vi "fgv_AOL Properties.vi"(8 "error in (no error)":errorcluster, 10 "Function":T2, 11 "AOL Properties in":T1={"AOD 1 thickness (mm)"=118.0, "AOD 2 thickness (mm)"=115.0, "AOD 3 thickness (mm)"=110.0, "AOD 4 thickness (mm)"=135.0, "AOD 5 thickness (mm)"=135.0, "AOD 6 thickness (mm)"=135.0, "AOD 1-2 separation (mm)"=15.0, "AOD 2-3 separation (mm)"=15.0, "AOD 3-4 separation (mm)"=15.0, "AOD 4-5 separation (mm)"=15.0, "AOD 5-6 separation (mm)"=15.0, "AOD 1 X Offset"=15.0, "AOD 2 X Offset"=1.0, "AOD 3 X Offset"=1.0, "AOD 4 X Offset"=1.0, "AOD 1 Y Offset"=1.0, "AOD 2 Y Offset"=1.0, "AOD 3 Y Offset"=1.0, "AOD 4 Y Offset"=1.0, "AOD 1 X Direction"=0.0, "AOD 2 X Direction"=0.0, "AOD 3 X Direction"=0.0, "AOD 4 X Direction"=0.0, "AOD 1 Y Direction"=1.0, "AOD 2 Y Direction"=0.0, "AOD 3 Y Direction"=0.0023, "AOD 4 Y Direction"=0.0046, "AOD 1 Centre (mm)"=15.0, "AOD 2 Centre (mm)"=50.0, "AOD 3 Centre (mm)"=50.0, "AOD 4 Centre (mm)"=50.0, "Timing Offset AOD 1"=0.0, "Timing Offset AOD 2"=0.0, "Timing Offset AOD 3"=0.0, "Timing Offset AOD 4"=0.0, "AOD Optical offset 1"=20000.0, "AOD Optical offset 2"=20000.0, "AOL aperture (mm)"=15.0, "AOL centre wavelength (nm)"=1.0, "AOL centre frequency (MHz)"=1.0, "Diffraction mode"=1.0, "Crystal length (mm)"=0.0, "Acoustic velocity (m/s)"=1.0, "Pair deflection ratio"=1.0, "AOD fill time (us)"=1.0, "AOD Ord. Refractive index"=2.22, "AOD ExtraOrd. Refractive index"=2.22}) -> (0 "error out":errorcluster, 3 "AOL Properties out":T1={"AOD 1 thickness (mm)"=118.0, "AOD 2 thickness (mm)"=115.0, "AOD 3 thickness (mm)"=110.0, "AOD 4 thickness (mm)"=135.0, "AOD 5 thickness (mm)"=135.0, "AOD 6 thickness (mm)"=135.0, "AOD 1-2 separation (mm)"=15.0, "AOD 2-3 separation (mm)"=15.0, "AOD 3-4 separation (mm)"=15.0, "AOD 4-5 separation (mm)"=15.0, "AOD 5-6 separation (mm)"=15.0, "AOD 1 X Offset"=15.0, "AOD 2 X Offset"=1.0, "AOD 3 X Offset"=1.0, "AOD 4 X Offset"=1.0, "AOD 1 Y Offset"=1.0, "AOD 2 Y Offset"=1.0, "AOD 3 Y Offset"=1.0, "AOD 4 Y Offset"=1.0, "AOD 1 X Direction"=0.0, "AOD 2 X Direction"=0.0, "AOD 3 X Direction"=0.0, "AOD 4 X Direction"=0.0, "AOD 1 Y Direction"=1.0, "AOD 2 Y Direction"=0.0, "AOD 3 Y Direction"=0.0023, "AOD 4 Y Direction"=0.0046, "AOD 1 Centre (mm)"=15.0, "AOD 2 Centre (mm)"=50.0, "AOD 3 Centre (mm)"=50.0, "AOD 4 Centre (mm)"=50.0, "Timing Offset AOD 1"=0.0, "Timing Offset AOD 2"=0.0, "Timing Offset AOD 3"=0.0, "Timing Offset AOD 4"=0.0, "AOD Optical offset 1"=20000.0, "AOD Optical offset 2"=20000.0, "AOL aperture (mm)"=15.0, "AOL centre wavelength (nm)"=1.0, "AOL centre frequency (MHz)"=1.0, "Diffraction mode"=1.0, "Crystal length (mm)"=0.0, "Acoustic velocity (m/s)"=1.0, "Pair deflection ratio"=1.0, "AOD fill time (us)"=1.0, "AOD Ord. Refractive index"=2.22, "AOD ExtraOrd. Refractive index"=2.22})   [LabVIEW 2017]
uses:
  Typedefs/AOL Properties Cluster.ctl
  Typedefs/HW config states enum.ctl
  Typedefs/Save-Load enum.ctl
  General Globals.vi
panel:
  # "FUNCTIONAL GLOBAL"
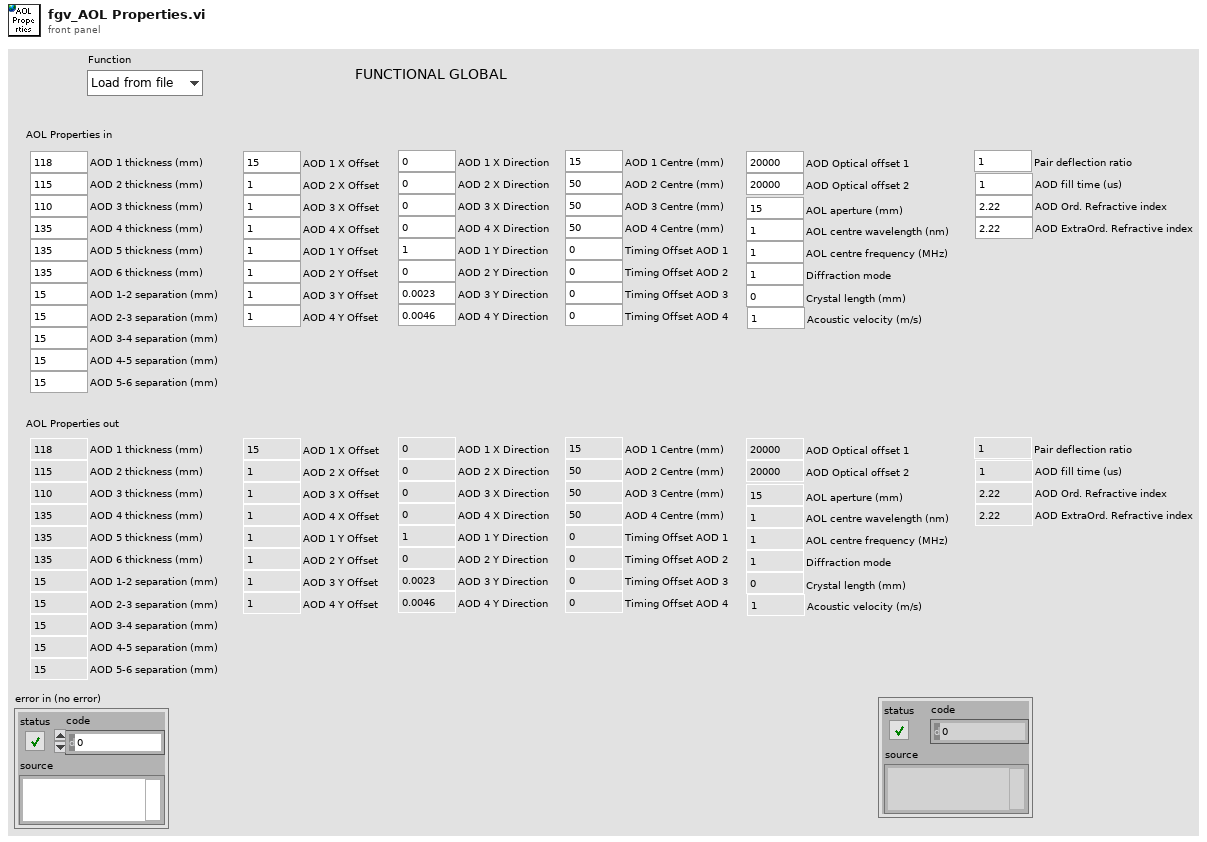
[diagram p1: front panel]
types:
  T1 = typedef "AOL Properties Cluster.ctl" = cluster{"AOD 1 thickness (mm)":dbl, "AOD 2 thickness (mm)":dbl, "AOD 3 thickness (mm)":dbl, "AOD 4 thickness (mm)":dbl, "AOD 5 thickness (mm)":dbl, "AOD 6 thickness (mm)":dbl, "AOD 1-2 separation (mm)":dbl, "AOD 2-3 separation (mm)":dbl, "AOD 3-4 separation (mm)":dbl, "AOD 4-5 separation (mm)":dbl, "AOD 5-6 separation (mm)":dbl, "AOD 1 X Offset":dbl, "AOD 2 X Offset":dbl, "AOD 3 X Offset":dbl, "AOD 4 X Offset":dbl, "AOD 1 Y Offset":dbl, "AOD 2 Y Offset":dbl, "AOD 3 Y Offset":dbl, "AOD 4 Y Offset":dbl, "AOD 1 X Direction":dbl, "AOD 2 X Direction":dbl, "AOD 3 X Direction":dbl, "AOD 4 X Direction":dbl, "AOD 1 Y Direction":dbl, "AOD 2 Y Direction":dbl, "AOD 3 Y Direction":dbl, "AOD 4 Y Direction":dbl, "AOD 1 Centre (mm)":dbl, "AOD 2 Centre (mm)":dbl, "AOD 3 Centre (mm)":dbl, "AOD 4 Centre (mm)":dbl, "Timing Offset AOD 1":dbl, "Timing Offset AOD 2":dbl, "Timing Offset AOD 3":dbl, "Timing Offset AOD 4":dbl, "AOD Optical offset 1":dbl, "AOD Optical offset 2":dbl, "AOL aperture (mm)":dbl, "AOL centre wavelength (nm)":dbl, "AOL centre frequency (MHz)":dbl, "Diffraction mode":dbl, "Crystal length (mm)":dbl, "Acoustic velocity (m/s)":dbl, "Pair deflection ratio":dbl, "AOD fill time (us)":dbl, "AOD Ord. Refractive index":dbl, "AOD ExtraOrd. Refractive index":dbl}
  T2 = typedef "HW config states enum.ctl" = enum16{"Load from file", "Save to file", "Write all", "Read all", "Write XY stage settings", "Write DAQ FPGA settings", "Write Control FPGA settings", "Write Phys Channels", "Clear", "Compare from file"}
  T3 = typedef "Save-Load enum.ctl" = enum16{"Save to file", "Load from file", "Compare from file"}
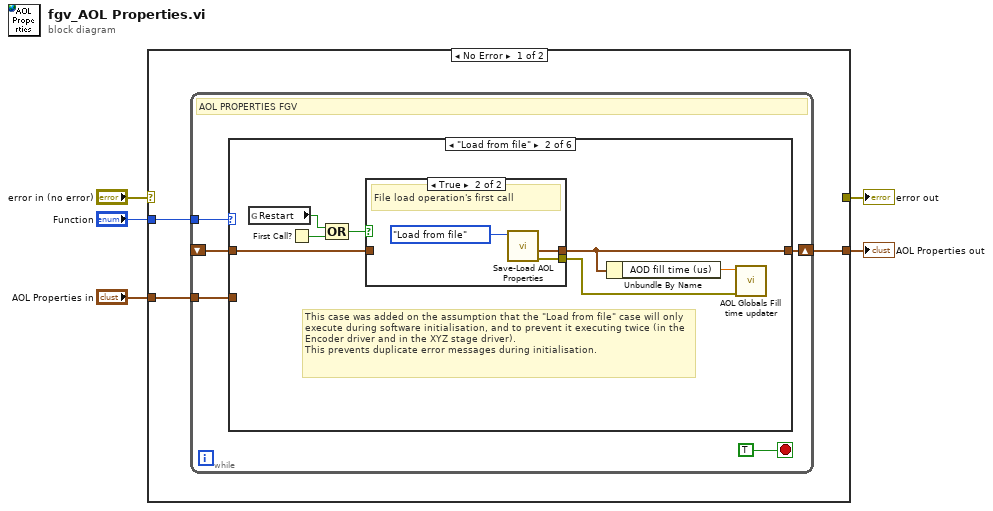
[diagram p0: block diagram]
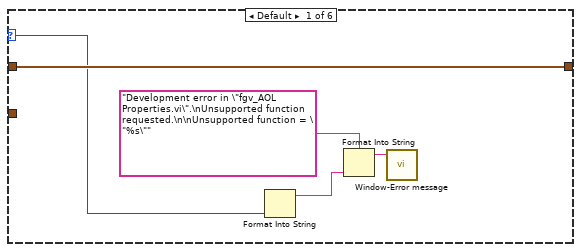
[diagram p2: hidden frame]
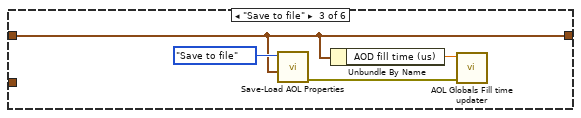
[diagram p4: hidden frame]
diagram:
  n1 = case shown="No Error" "error in (no error)" {
    selector: "error in (no error)" -> [_ w36]
    tunnel: [_ w36] -> w4
    tunnel: "Function" -> [w8 _]
    tunnel: "AOL Properties in" -> [w7 _]
    tunnel: [w6 _] -> w1
    frame No Error {
      n2 = while {
        tunnel: w8 -> [w13]
        shift-right: [w11] -> w6
        shift-left: _ -> [w9]
        tunnel: w7 -> [w10]
        stop <- TRUE stop-if-true
        # "AOL PROPERTIES FGV"
        n3 = case shown="\"Load from file\"" w13 {
          selector: w13 -> [w14 _ _ _ _ _]
          tunnel: [w15 w24 w31 w34 w35 _] -> w11
          tunnel: w10 -> [_ _ _ w34 _ _]
          tunnel: w9 -> [w15 w25 w31 _ w35 _]
          frame Default {
            n4 = Format Into String(w14) -> (resulting string=w17:string)  [unwired: 3 in, 1 out]
            n5 = Format Into String(format string="Development error in \"fgv_AOL Properties.vi\".\nUnsupported function requested.\n\nUnsupported function = \"%s\"" ("Message"), w17) -> (resulting string=w16:string)  [unwired: 2 in, 1 out]
            n6 = call "Window-Error message.vi"("Message"=w16) -> ()  [unwired: 10 in, 1 out]
          }
          frame "Load from file" {
            # "This case was added on the assumption that the \"Load from file\" case will only execute during software initialisation, and to prevent it executing twice (in the Encoder driver and in the XYZ stage driver).\nThis prevents duplicate error messages during initialisation."
            n7 = global read "General Globals.vi" "Restart"() -> (w20:bool)
            n8 = First Call?() -> (First Call?: T/F=w21:bool)
            n9 = Compound Arithmetic op=OR(w20, w21) -> (w19:bool)
            n10 = case shown="True" w19 {
              tunnel: [w26 w28] -> w24
              tunnel: w25 -> [w26 _]
              tunnel: [_ w27] -> w23
              frame False {
                # "Already loaded"
              }
              frame True {
                # "File load operation's first call"
                n11 = call "Save-Load AOL Properties.vi"("Function"=Save-Load_enum."Load from file") -> ("error out"=w27:errorcluster, "AOL Properties OUT"=w28:T1)  [unwired: 9 in]
              }
            }
            n12 = Unbundle By Name(w24) -> ("AOD fill time (us)"=w22:dbl)
            n13 = call "AOL Globals Fill time updater.vi"("error in"=w23, "AOD fill time (us)"=w22) -> ()  [unwired: 9 in, 1 out]
          }
          frame "Save to file" {
            n14 = call "Save-Load AOL Properties.vi"("AOL Properties IN"=w31, "Function"=Save-Load_enum."Save to file") -> ("error out"=w32:errorcluster)  [unwired: 8 in, 1 out]
            n15 = Unbundle By Name(w31) -> ("AOD fill time (us)"=w30:dbl)
            n16 = call "AOL Globals Fill time updater.vi"("error in"=w32, "AOD fill time (us)"=w30) -> ()  [unwired: 9 in, 1 out]
          }
          frame "Write all" {
          }
          frame "Read all" {
          }
          frame "Clear" {
          }
        }
      }
    }
    frame Error {
    }
  }
  "error out" <- w4
  "AOL Properties out" <- w1
